vi "Hatch Mover Immediate.vi"(7 "Description":string, 8 "Command Info In":T1, 9 "Deadband Value":dbl=0.01, 11 "Setpoint":dbl) -> (0 "Command Info Out":T1)   [LabVIEW 2018]
doc: "This template is useful for immediate subsystem actions that do not need deadband filtering\n\nBe sure to right-click and select New from Template and save with a new command name."
uses:
  <vilib>/Rock Robotics/WPI/Framework/Command Status Info.ctl
  <vilib>/Rock Robotics/WPI/Framework/Completion Status.ctl
  <vilib>/Rock Robotics/WPI/Framework/Completion Notifier.ctl
  Implementation/Hatch Mover Setpoints.ctl
  Implementation/Hatch Mover Operations.ctl
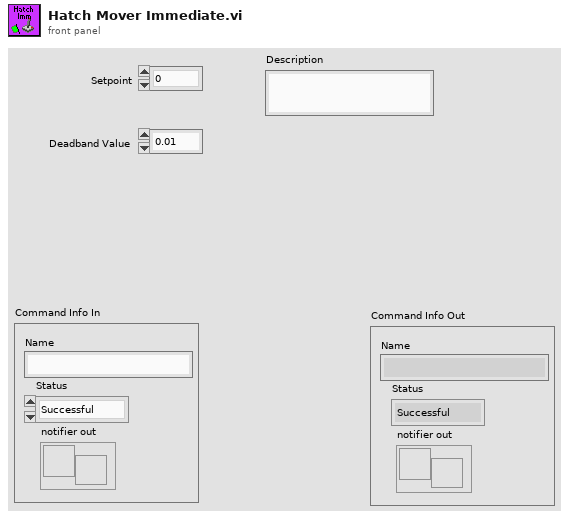
[diagram p1: front panel]
types:
  T1 = typedef "Command Status Info.ctl" = cluster{"Name":string, "Status":T2, "notifier out":T3}
  T2 = typedef "Completion Status.ctl" = enum16{"Successful", "Aborted", "Incomplete"}
  T3 = typedef "Completion Notifier.ctl" = refnum<notifier>
  T4 = typedef "Hatch Mover Setpoints.ctl" = cluster{"Operation":T5, "Setpoint":dbl, "Duration":dbl}
  T5 = typedef "Hatch Mover Operations.ctl" = enum16{"Reserve", "Read Current", "Immediate", "Extend", "Retract"}
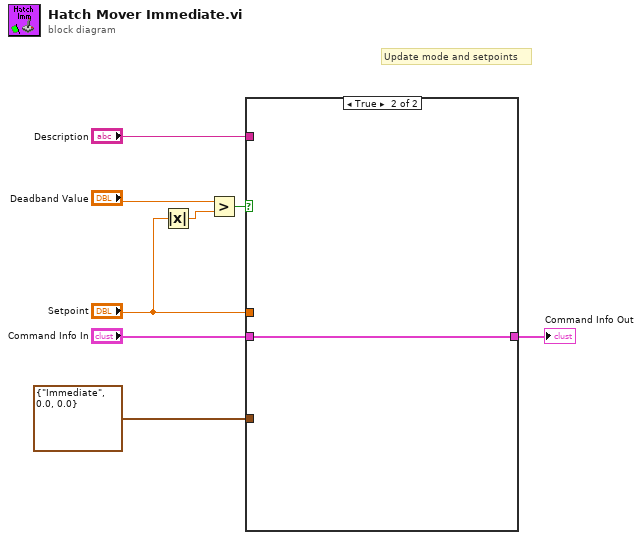
[diagram p0: block diagram]
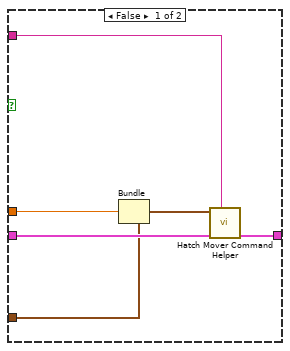
[diagram p2: hidden frame]
diagram:
  # "Update mode and setpoints"
  n1 = Absolute Value(x="Setpoint") -> (abs(x)=w4:dbl)
  n2 = Greater?(x="Deadband Value", y=w4) -> (0:w1:bool)
  n3 = case shown="True" w1 {
    tunnel: [w14 w15] -> w8
    tunnel: "Command Info In" -> [w13 w15]
    tunnel: "Description" -> [w12 _]
    tunnel: T4 {"Operation"=enum."Immediate", "Setpoint"=0.0, "Duration"=0.0} ("SubSystem Data") -> [w11 _]
    tunnel: "Setpoint" -> [w10 _]
    frame False {
      n4 = Bundle(cluster=w11, "Setpoint"=w10) -> (w9:T4)  [unwired: 2 in]
      n5 = call "Hatch Mover Command Helper.vi"("Description"=w12, "Command Info In"=w13, "SubSystem Data"=w9) -> ("Command Info Out"=w14:T1)  [unwired: 6 in, 2 out]
    }
    frame True {
    }
  }
  "Command Info Out" <- w8
